vi "Normalized Case.vi"(0 "m":u32[](array[numeric]), 1 "n-m":u32[](array[numeric]), 2 "table":dbl[][](array[numeric]) format="%.2f") -> (3 "m*":u32[](array[numeric]), 4 "n-m*":u32[](array[numeric]), 5 "table*":dbl[][](array[numeric]) format="%.2f", 6 "error":i32)   [LabVIEW 2018, in "NI_Gmath.lvlib"]
uses:
  NI_Gmath.lvlib
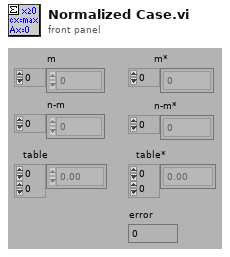
[diagram p1: front panel]
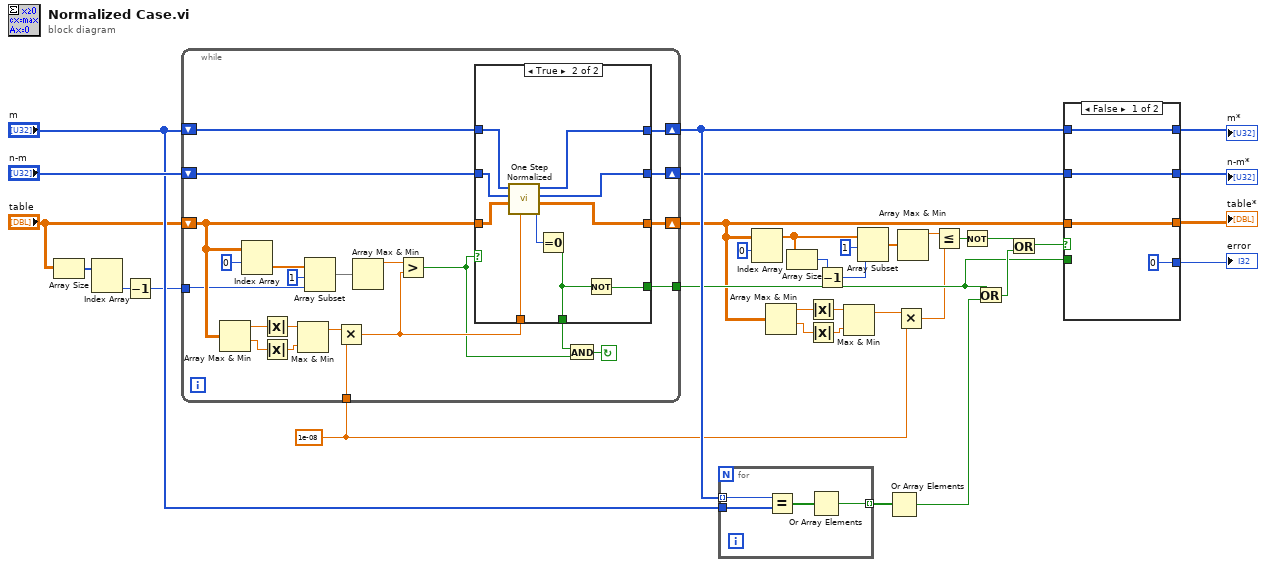
[diagram p0: block diagram]
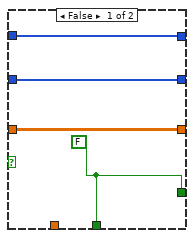
[diagram p2: hidden frame]
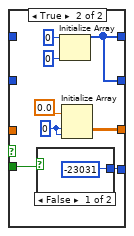
[diagram p3: hidden frame]
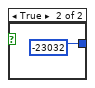
[diagram p4: hidden frame]
diagram:
  w12 = 1e-08
  n1 = Array Size(array="table") -> (size(s)=w3:i32[])
  n2 = Index Array(array=w3) -> (element #2=w2:i32)  [unwired: 2 in, 1 out]
  n3 = Decrement(x=w2) -> (x-1=w1:i32)
  n4 = while {
    tunnel: w12 -> [w49]
    tunnel: [w53] -> w14
    shift-left: "table" -> [w45]
    shift-right: [w52] -> w6
    shift-left: "n-m" -> [w56]
    shift-right: [w50] -> w29
    shift-left: "m" -> [w57]
    shift-right: [w51] -> w31
    tunnel: w1 -> [w38]
    stop <- w54 continue-if-true
    n5 = Array Max & Min(array=w45) -> (max value=w41:dbl, min value=w42:dbl)  [unwired: 2 out]
    n6 = Index Array(array=w45, index (row)=0) -> (element=w39:dbl[])  [unwired: 1 in]
    n7 = Absolute Value(x=w41) -> (abs(x)=w43:dbl)
    n8 = Absolute Value(x=w42) -> (abs(x)=w44:dbl)
    n9 = Max & Min(x=w43, y=w44) -> (max(x,y)=w47:dbl)  [unwired: 1 out]
    n10 = Array Subset(array=w39, index=1, length=w38) -> (w36:dbl[])
    n11 = Multiply(x=w47, y=w49) -> (x*y=w48:dbl)
    n12 = Array Max & Min(array=w36) -> (max value=w35:dbl)  [unwired: 3 out]
    n13 = Greater?(x=w35, y=w48) -> (0:w37:bool)
    n14 = case shown="True" w37 {
      tunnel: w57 -> [w61 w70]
      tunnel: [w61 w64] -> w51
      tunnel: w45 -> [w60 w68]
      tunnel: [w60 w62] -> w52
      tunnel: w56 -> [w59 w69]
      tunnel: [w59 w63] -> w50
      tunnel: [w58 w67] -> w55
      tunnel: [w58 w66] -> w53
      tunnel: w48 -> [_ w65]
      frame False {
        w58 = FALSE
      }
      frame True {
        n15 = call "One Step Normalized.vi"("eps"=w65, "table"=w68, "n-m"=w69, "m"=w70) -> ("error"=w71:i32, "table*"=w62:dbl[][], "n-m*"=w63:u32[], "m*"=w64:u32[])  [unwired: 4 in]
        n16 = Equal To 0?(x=w71) -> (x = 0?=w67:bool)
        n17 = Not(x=w67) -> (.not. x?=w66:bool)
      }
    }
    n18 = And(x=w55, y=w37) -> (x .and. y?=w54:bool)
  }
  n19 = for {
    tunnel: w31 -> [w75] mode=indexing
    tunnel: "m" -> [w74]
    tunnel: [w72] -> w32 mode=indexing
    n20 = Equal?(x=w75, y=w74) -> (x = y?=w73:bool[])
    n21 = Or Array Elements(Boolean array=w73) -> (logical OR=w72:bool)
  }
  n22 = Index Array(array=w6, index (row)=0) -> (element=w23:dbl[])  [unwired: 1 in]
  n23 = Array Max & Min(array=w6) -> (max value=w10:dbl, min value=w9:dbl)  [unwired: 2 out]
  n24 = Array Size(array=w23) -> (size(s)=w22:i32)
  n25 = Absolute Value(x=w10) -> (abs(x)=w8:dbl)
  n26 = Absolute Value(x=w9) -> (abs(x)=w7:dbl)
  n27 = Decrement(x=w22) -> (x-1=w21:i32)
  n28 = Max & Min(x=w8, y=w7) -> (max(x,y)=w5:dbl)  [unwired: 1 out]
  n29 = Array Subset(array=w23, index=1, length=w21) -> (w20:dbl[])
  n30 = Or Array Elements(Boolean array=w32) -> (logical OR=w13:bool)
  n31 = Multiply(x=w5, y=w12) -> (x*y=w11:dbl)
  n32 = Array Max & Min(array=w20) -> (max value=w16:dbl)  [unwired: 3 out]
  n33 = Less Or Equal?(x=w16, y=w11) -> (x <= y?=w19:bool)
  n34 = Not(x=w19) -> (.not. x?=w15:bool)
  n35 = Or(x=w14, y=w13) -> (x .or. y?=w18:bool)
  n36 = Or(x=w15, y=w18) -> (x .or. y?=w17:bool)
  n37 = case shown="False" w17 {
    tunnel: w31 -> [w79 _]
    tunnel: [w79 w85] -> w30
    tunnel: w29 -> [w78 _]
    tunnel: [w78 w85] -> w28
    tunnel: [0 w87] -> w27
    tunnel: [w76 w81] -> w26
    tunnel: w6 -> [w76 _]
    tunnel: w14 -> [_ w80]
    frame False {
    }
    frame True {
      w83 = 0
      n38 = case shown="False" w80 {
        tunnel: [-23031 -23032] -> w87
        frame False {
        }
        frame True {
        }
      }
      n39 = Initialize Array(u32 0, 0) -> (w85:u32[])
      n40 = Initialize Array(0.0, w83, w83) -> (w81:dbl[][])
    }
  }
  "n-m*" <- w28
  "m*" <- w30
  "error" <- w27
  "table*" <- w26
